vi "vi01_PID_gain_conversion.vi"() -> ()   [LabVIEW 2025]
panel:
  in  "Ts":dbl format="%#_6p"
  out "Kd":dbl
  out "Ki":dbl
  in  "Td":dbl
  in  "Ti":dbl
  out "Kp":dbl
  in  "Kc":dbl
  # "PID Gain Conversion: Discrete to Continuous"
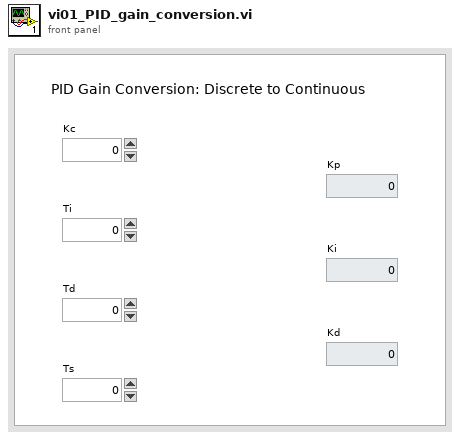
[diagram p1: front panel]
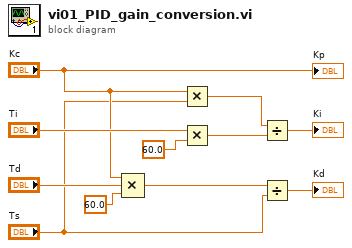
[diagram p0: block diagram]
diagram:
  n1 = Compound Arithmetic op=MULTIPLY("Kc", "Td", 60.0 ("value")) -> (w3:dbl)
  n2 = Multiply(x="Kc", y="Ts") -> (x*y=w8:dbl)
  n3 = Multiply(x="Ti", y=60.0) -> (x*y=w7:dbl)
  n4 = Divide(x=w8, y=w7) -> (x/y=→"Ki":dbl)
  n5 = Divide(x=w3, y="Ts") -> (x/y=→"Kd":dbl)
  "Kp" <- "Kc"
